vi "Get Multi Numeric.vi"(6 "Write?":bool, 8 "error in (no error)":errorcluster, 9 "Tag":string[](array[string]), 10 "Value Type":refnum<class "Abs_Numeric.lvclass">[](array[class]), 11 "Var Bus in":refnum<class "Omni_Bus.lvclass">) -> (0 "error out":errorcluster, 2 "Value Out":refnum<class "Abs_Numeric.lvclass">[](array[class]), 3 "Var Bus out":refnum<class "Omni_Bus.lvclass">)   [LabVIEW 2021, in "Omni_Bus.lvclass"]
uses:
  Omni_Bus.lvclass
  Omni_Bus.lvclass/Omni_Bus.ctl
  <vilib>/TSA/Abstract Data Classes/Abs_Types/Numeric/Abs_Numeric.lvclass
  C:/Program Files (x86)/National Instruments/LabVIEW 2021/vi.lib/TSA/Abstract Data Classes/Abs_Types/Value/Abs_Value.lvclass
  C:/Program Files (x86)/National Instruments/LabVIEW 2021/vi.lib/TSA/Abstract Data Classes/Abs_Types/Type/Abs_Type.lvclass
  C:/Program Files (x86)/National Instruments/LabVIEW 2021/vi.lib/TSA/Abstract Data Classes/Abs_Types/Numeric/Abs_Numeric.lvclass
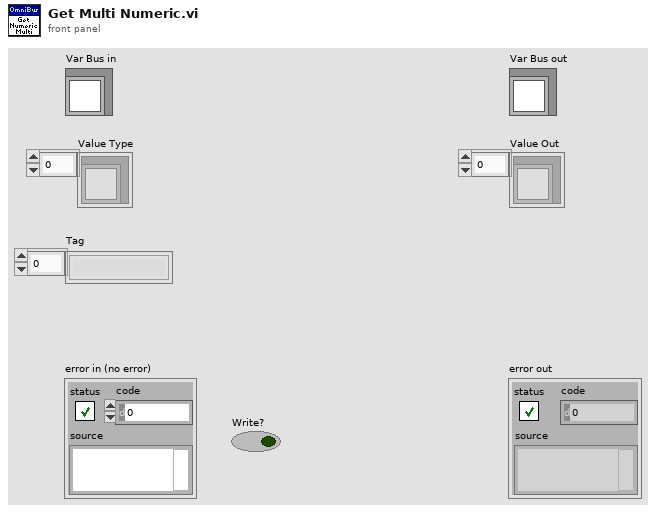
[diagram p1: front panel]
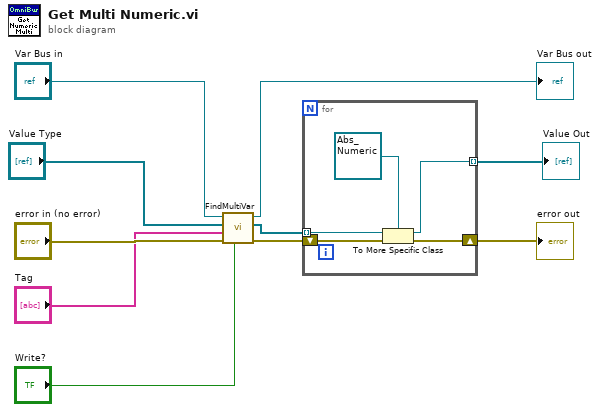
[diagram p0: block diagram]
diagram:
  n1 = call "FindMultiVar.vi"("Write?"="Write?", "error in (no error)"="error in (no error)", "Tag"="Tag", "Abs_Type Default"="Value Type", "Var Bus in"="Var Bus in") -> ("error out"=w7:errorcluster, "Abs_Type Found"=w6:refnum<class "Abs_Type.lvclass">[], "Var Bus out"=→"Var Bus out":refnum<class "Omni_Bus.lvclass">)  [unwired: 4 in]
  n2 = for {
    tunnel: w6 -> [w14] mode=indexing
    tunnel: [w11] -> w2 mode=indexing
    shift-right: [w13] -> w4
    shift-left: w7 -> [w15]
    n3 = To More Specific Class(target class=refnum<class "Abs_Numeric.lvclass"> refnum ("Abs_Numeric.lvclass out"), reference=w14, error in=w15) -> (specific class reference=w11:refnum<class "Abs_Numeric.lvclass">, error out=w13:errorcluster)
  }
  "error out" <- w4
  "Value Out" <- w2
